vi "LR-Stabilization-time.vi"(5 "Test characteristics":T2, 7 "Stabilization time settings":T4={"Max. delta [%]"=80, "Min. segment length"=0}, 8 "error in (no error)":errorcluster, 9 "Power in":dbl[](array[numeric]), 11 "Results in":T1) -> (0 "error out":errorcluster, 1 "Power":dbl[](array[numeric]), 3 "Results":T1, 4 "Valid?":bool)   [LabVIEW 2013, in "HardwareCharacterization.lvlib" / "HC-LaserResponse.lvclass"]
doc: "Use this template to build a VI to use as a subVI."
uses:
  HC-LaserResponse.lvclass
  Settings-stabilization.ctl
  Test-characteristics.ctl
  Detectors.ctl
  Test-results.ctl
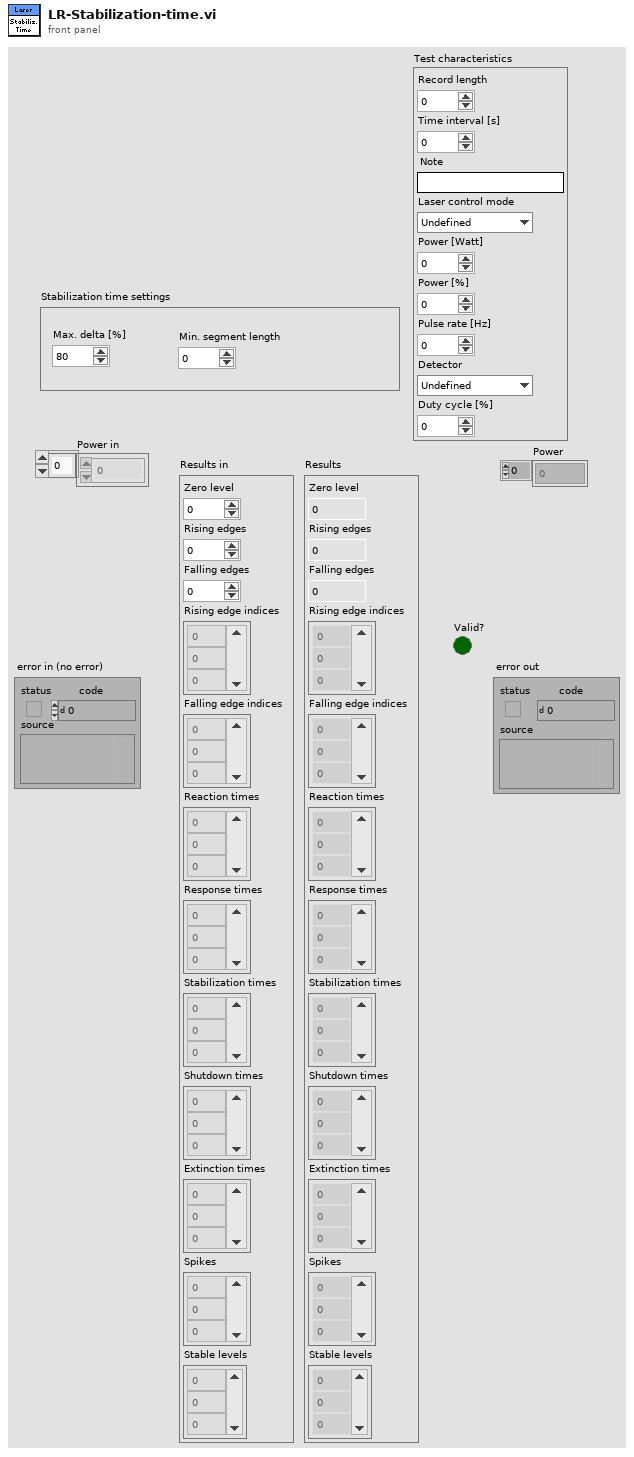
[diagram p1: front panel]
types:
  T1 = typedef "HardwareCharacterization.lvlib/HC-LaserResponse.lvclass/Test-results.ctl" = cluster{"Zero level":dbl, "Rising edges":i32, "Falling edges":i32, "Rising edge indices":dbl[], "Falling edge indices":dbl[], "Reaction times":dbl[], "Response times":dbl[], "Stabilization times":dbl[], "Shutdown times":dbl[], "Extinction times":dbl[], "Spikes":i32[], "Stable levels":dbl[]}
  T2 = typedef "HardwareCharacterization.lvlib/HC-LaserResponse.lvclass/Test-characteristics.ctl" = cluster{"Record length":i32, "Time interval [s]":dbl, "Note":string, "Laser control mode":enum16{"Undefined", "Modulation (digital)", "Power variation (analog)"}, "Power [Watt]":dbl, "Power [%]":dbl, "Pulse rate [Hz]":dbl, "Detector":T3, "Duty cycle [%]":dbl}
  T3 = typedef "HardwareCharacterization.lvlib/HC-LaserResponse.lvclass/Detectors.ctl" = enum16{"Undefined", "DET10A", "DET10A - 2kOhm ", "PDA36A - 0dB"}
  T4 = typedef "HardwareCharacterization.lvlib/HC-LaserResponse.lvclass/Settings-stabilization.ctl" = cluster{"Max. delta [%]":i32, "Min. segment length":i32}
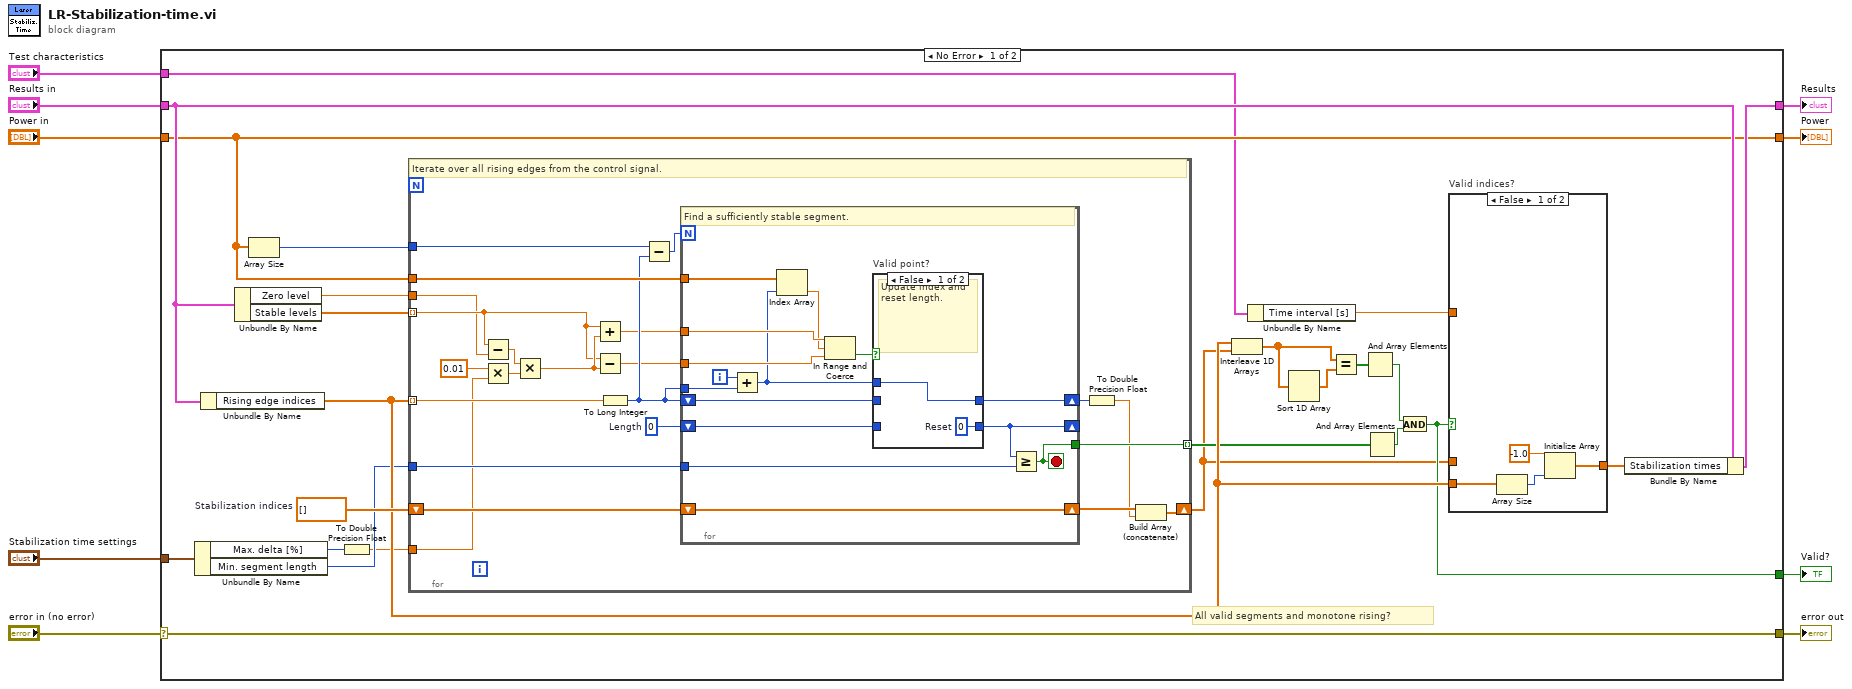
[diagram p0: block diagram]
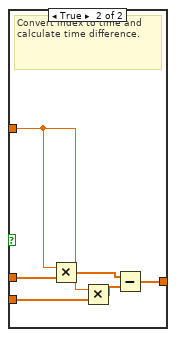
[diagram p2: hidden frame]
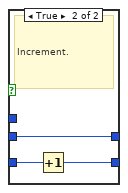
[diagram p3: hidden frame]
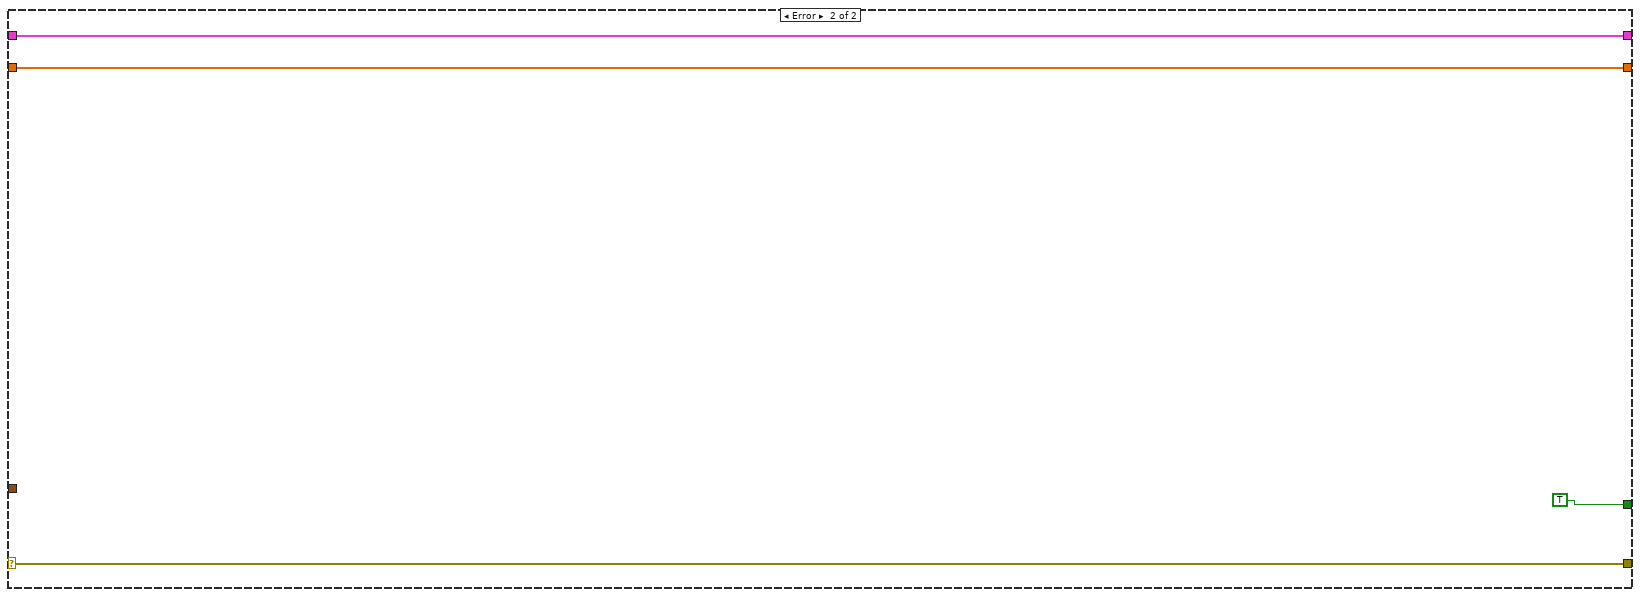
[diagram p4: hidden frame]
diagram:
  n1 = case shown="No Error" "error in (no error)" {
    selector: "error in (no error)" -> [w31 w89]
    tunnel: [w31 w89] -> w8
    tunnel: "Results in" -> [w26 w88]
    tunnel: "Stabilization time settings" -> [w33 _]
    tunnel: [w23 TRUE] -> w7
    tunnel: [w27 w88] -> w3
    tunnel: "Power in" -> [w16 w86]
    tunnel: [w16 w86] -> w2
    tunnel: "Test characteristics" -> [w15 _]
    frame No Error {
      w32 = dbl[] []  # Stabilization indices
      # "All valid segments and monotone rising?"
      n2 = Unbundle By Name(w33) -> ("Max. delta [%]"=w13:i32, "Min. segment length"=w20:i32)
      n3 = Unbundle By Name(w26) -> ("Rising edge indices"=w24:dbl[])
      n4 = Unbundle By Name(w26) -> ("Zero level"=w11:dbl, "Stable levels"=w10:dbl[])
      n5 = Array Size(array=w16) -> (size(s)=w21:i32)
      n6 = To Double Precision Float(number=w13) -> (double precision float=w12:dbl)
      n7 = for {
        tunnel: w16 -> [w61]
        tunnel: w24 -> [w55] mode=indexing
        shift-right: [w57] -> w17
        shift-left: w32 -> [w63]
        tunnel: w21 -> [w65]
        tunnel: w20 -> [w62]
        tunnel: [w56] -> w19 mode=indexing
        tunnel: w12 -> [w46]
        tunnel: w11 -> [w44]
        tunnel: w10 -> [w45] mode=indexing
        w60 = 0  # Length
        # "Iterate over all rising edges from the control signal."
        n8 = Subtract(x=w45, y=w44) -> (x-y=w50:dbl)
        n9 = Multiply(x=0.01, y=w46) -> (x*y=w51:dbl)
        n10 = Multiply(x=w50, y=w51) -> (x*y=w49:dbl)
        n11 = Add(x=w45, y=w49) -> (x+y=w48:dbl)
        n12 = Subtract(x=w45, y=w49) -> (x-y=w47:dbl)
        n13 = To Long Integer(number=w55) -> (32bit integer=w54:i32)
        n14 = Subtract(x=w65, y=w54) -> (x-y=w64:i32)
        n15 = for {
          N: w64 -> [_]
          shift-right: [w75] -> _
          shift-left: w60 -> [w78]
          tunnel: w62 -> [w76]
          tunnel: w47 -> [w80]
          shift-right: [w77] -> w58
          shift-left: w54 -> [w68]
          tunnel: [w74] -> w56
          shift-right: [w67] -> w59
          shift-left: w63 -> [w67]
          tunnel: w61 -> [w72]
          tunnel: w48 -> [w73]
          tunnel: w54 -> [w66]
          i -> [w69]
          stop <- w74 stop-if-true
          # "Find a sufficiently stable segment."
          n16 = Add(x=w69, y=w66) -> (x+y=w70:i32)
          n17 = Index Array(array=w72, index=w70) -> (element=w71:dbl)
          n18 = In Range and Coerce(upper limit=w73, x=w71, lower limit=w80) -> (In Range?=w79:bool)  [unwired: 1 out]
          n19 = case "Valid point?" shown="False" w79 {
            tunnel: w78 -> [_ w85]
            tunnel: [w82 w84] -> w75
            tunnel: w70 -> [w81 _]
            tunnel: [w81 w83] -> w77
            tunnel: w68 -> [_ w83]
            frame False {
              w82 = 0  # Reset
              # "Update index and reset length."
            }
            frame True {
              # "Increment."
              n20 = Increment(x=w85) -> (x+1=w84:i32)
            }
          }
          n21 = Greater Or Equal?(x=w75, y=w76) -> (x >= y?=w74:bool)
        }
        n22 = To Double Precision Float(number=w58) -> (double precision float=w53:dbl)
        n23 = Build Array (concatenate)(w59, w53) -> (w57:dbl[])
      }
      n24 = Interleave 1D Arrays(w24, w17) -> (w30:dbl[])
      n25 = Unbundle By Name(w15) -> ("Time interval [s]"=w14:dbl)
      n26 = Sort 1D Array(array=w30) -> (sorted array=w29:dbl[])
      n27 = Equal?(x=w30, y=w29) -> (x = y?=w28:bool[])
      n28 = And Array Elements(Boolean array=w28) -> (logical AND=w25:bool)
      n29 = And Array Elements(Boolean array=w19) -> (logical AND=w18:bool)
      n30 = And(x=w25, y=w18) -> (x .and. y?=w23:bool)
      n31 = case "Valid indices?" shown="False" w23 {
        tunnel: w17 -> [_ w40]
        tunnel: w24 -> [w36 w39]
        tunnel: [w34 w41] -> w22
        tunnel: w14 -> [_ w38]
        frame False {
          n32 = Array Size(array=w36) -> (size(s)=w35:i32)
          n33 = Initialize Array(-1.0, w35) -> (w34:dbl[])
        }
        frame True {
          # "Convert index to time and calculate time difference."
          n34 = Multiply(x=w38, y=w40) -> (x*y=w42:dbl[])
          n35 = Multiply(x=w38, y=w39) -> (x*y=w43:dbl[])
          n36 = Subtract(x=w42, y=w43) -> (x-y=w41:dbl[])
        }
      }
      n37 = Bundle By Name(cluster=w26, "Stabilization times"=w22) -> (w27:T1)
    }
    frame Error {
    }
  }
  "error out" <- w8
  "Valid?" <- w7
  "Power" <- w2
  "Results" <- w3
